vi "Do_Every_minute.vi"(1 "Ch Names":string[](array[string]), 2 "Values":dbl[](array[numeric]) format="%.2f") -> ()   [LabVIEW 2011]
uses:
  Do_Every_5mins.ctl
  Anemometry/Anemometry Sub Vis/Controls/In_Range.ctl
  ADAM Client/Sub VIs/ADAM Controls/Traverse_Level_State.ctl
  ADAM Client/Sub VIs/ADAM Controls/Valco_valve_ph.ctl
  ADAM_Global.vi
panel:
  out "Case":T1
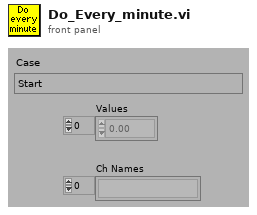
[diagram p1: front panel]
types:
  T1 = typedef "Do_Every_5mins.ctl" = enum16{"Start", "Update EnFlo Tunnel Speed Tweak", "Update Aero Tunnel Speed Tweak", "Aero Tunnel Server not live", "Are EnFlo Tun Fan Bearings too Hot?", "Check EnFlo tweak factor?", "Are Inlet Screens Blocked?", "Tweak demanded chilled water temp", "Is Dew point meter Alive?", "Condensation Occurring", "Condensation Alert", "More checks", "Set FFID Valve to Measure", "End"}
  T2 = typedef "In_Range.ctl" = enum16{"%", "±", "% & ±"}
  T3 = typedef "Traverse_Level_State.ctl" = enum16{"Running", "Complete"}
  T4 = typedef "Client_State_Cluster.ctl" = cluster{"Client Name":string, "Traverse level State":T3, "People to Email":string[], "Next Contact Time":dbl}
  T5 = typedef "Valco_valve_ph.ctl" = u16
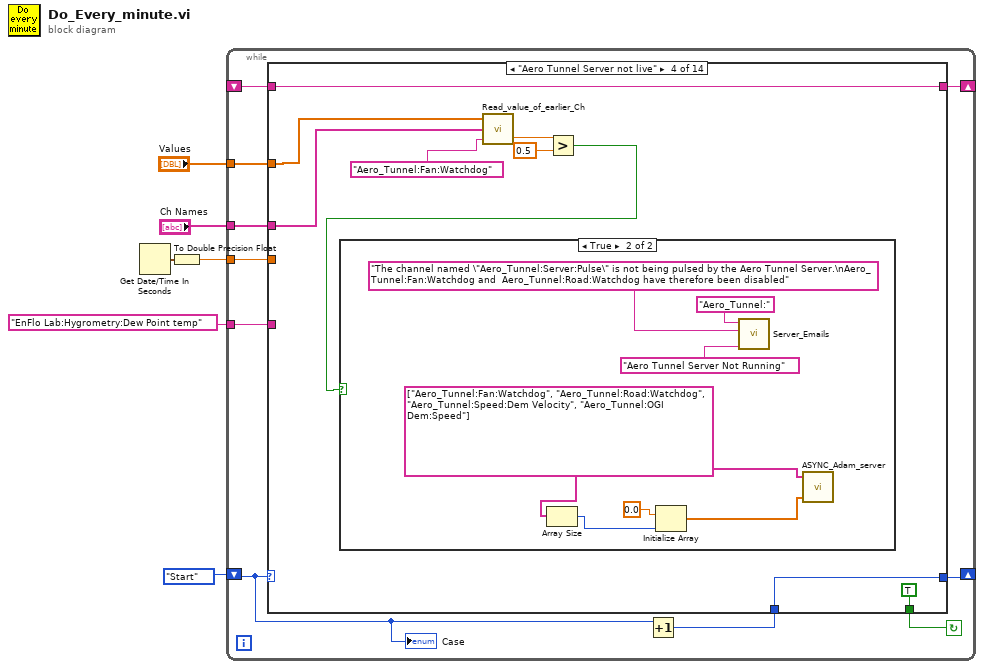
[diagram p0: block diagram]
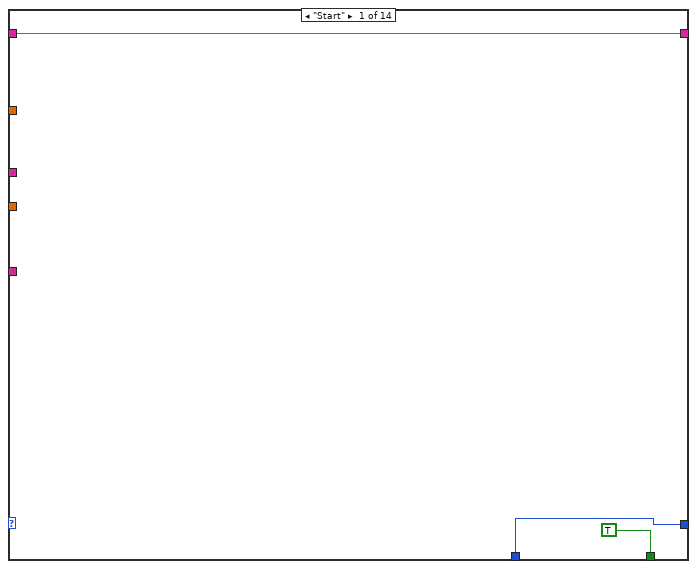
[diagram p2: hidden frame]
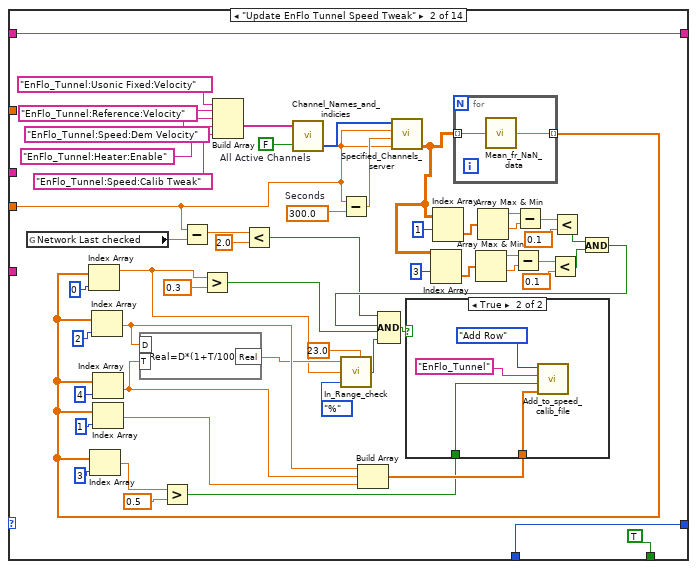
[diagram p3: hidden frame]
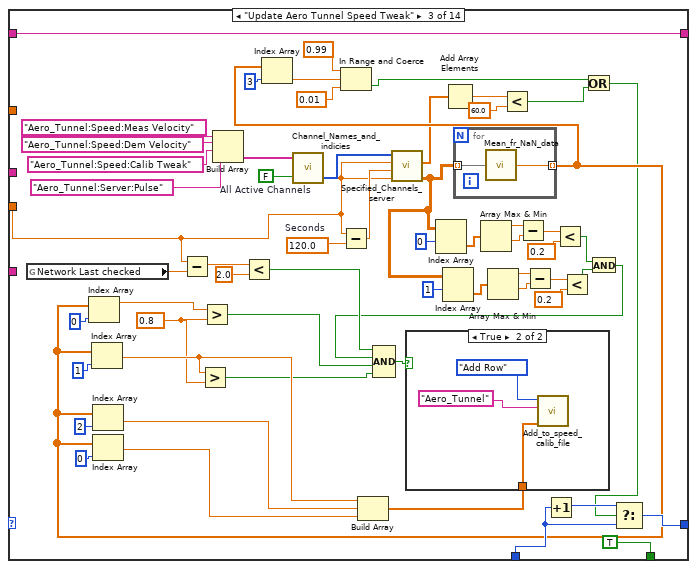
[diagram p5: hidden frame]
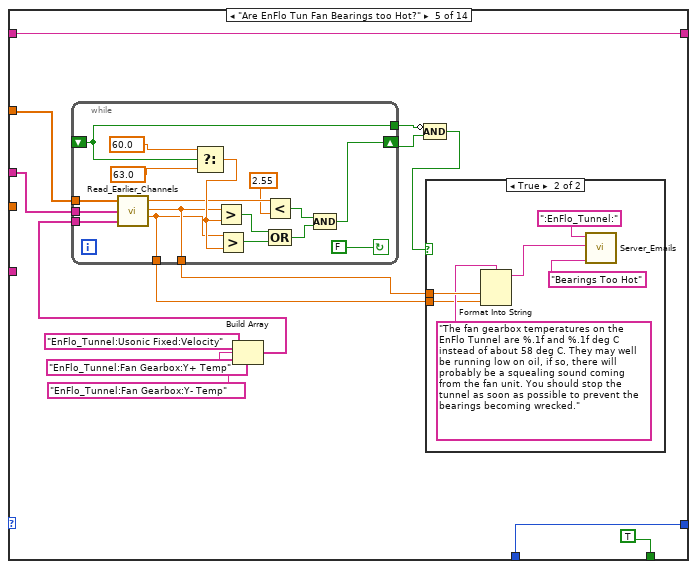
[diagram p8: hidden frame]
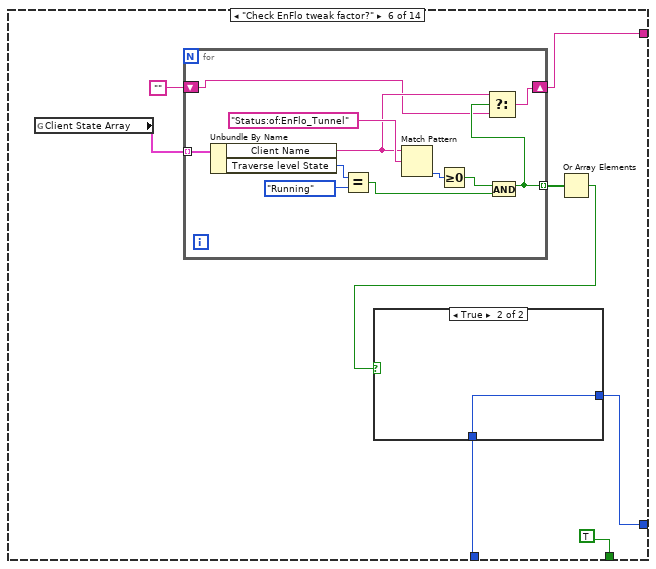
[diagram p10: hidden frame]
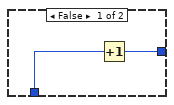
[diagram p11: hidden frame]
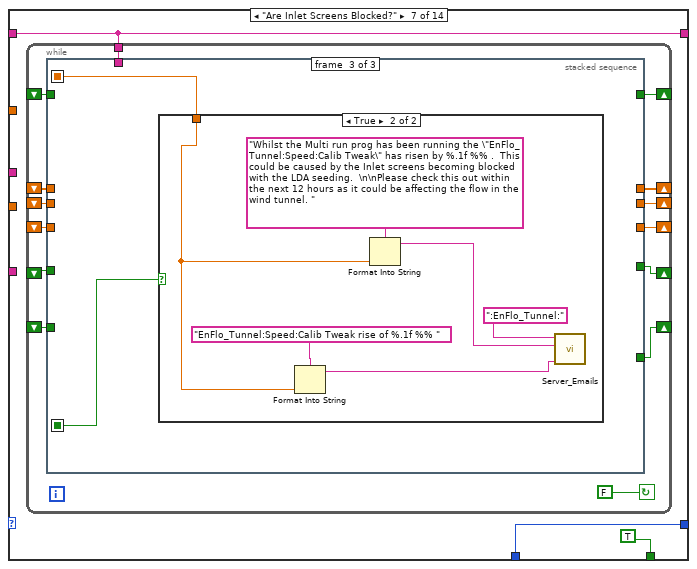
[diagram p12: hidden frame]
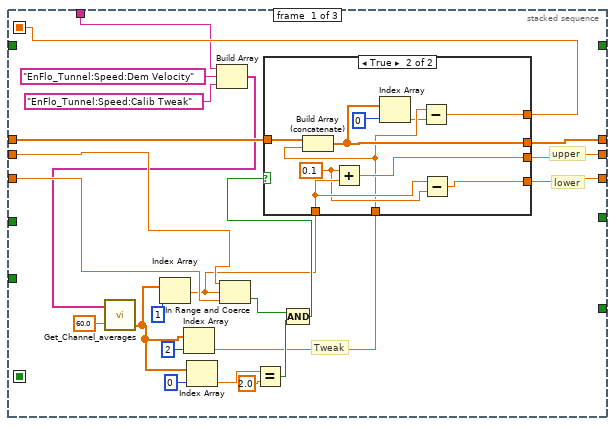
[diagram p13: hidden frame]
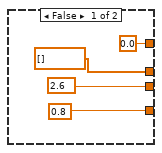
[diagram p14: hidden frame]
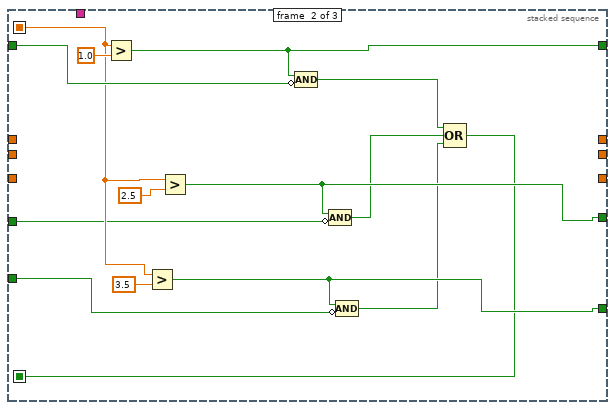
[diagram p15: hidden frame]
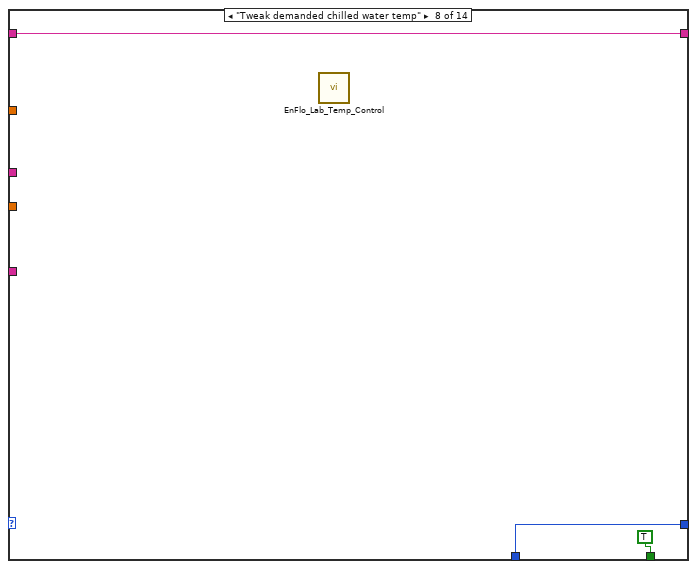
[diagram p17: hidden frame]
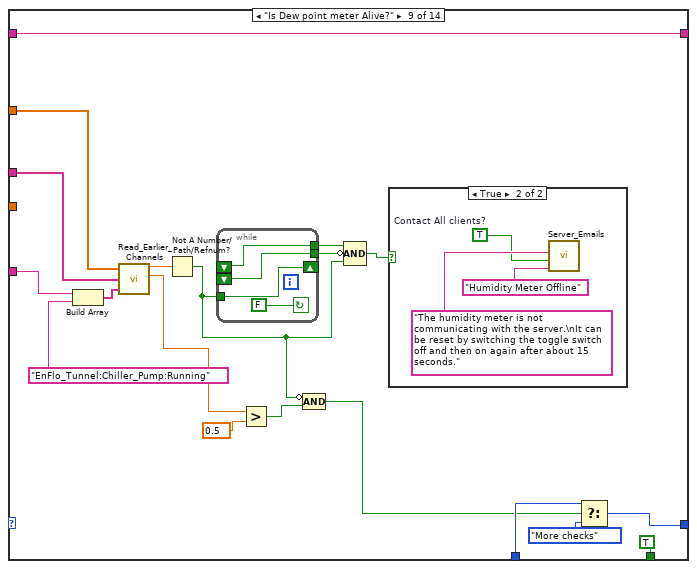
[diagram p18: hidden frame]
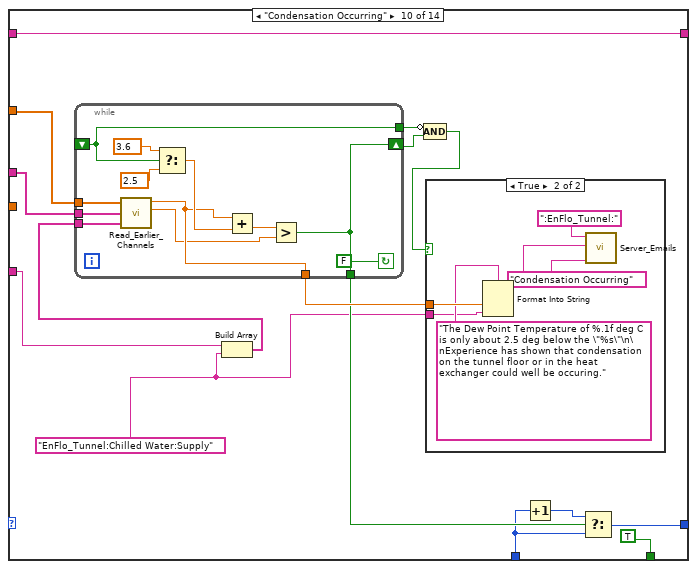
[diagram p20: hidden frame]
diagram:
  n1 = Get Date/Time In Seconds() -> (seconds since 1Jan1904=w2:timestamp)
  n2 = To Double Precision Float(number=w2) -> (double precision float=w1:dbl)
  n3 = while {
    tunnel: "EnFlo Lab:Hygrometry:Dew Point temp" -> [w10]
    tunnel: "Values" -> [w14]
    tunnel: "Ch Names" -> [w15]
    shift-left: Do_Every_5mins."Start" ("Case") -> [w11]
    shift-right: [w12] -> _
    tunnel: w1 -> [w9]
    shift-right: [w8] -> _
    shift-left: _ -> [w7]
    stop <- w16 continue-if-true
    n4 = Increment(x=w11) -> (x+1=w13:T1)
    n5 = case shown="\"Aero Tunnel Server not live\"" w11 {
      tunnel: [TRUE TRUE TRUE TRUE TRUE TRUE TRUE TRUE TRUE TRUE TRUE TRUE TRUE FALSE] -> w16
      tunnel: w15 -> [_ _ _ w148 w171 _ _ _ w313 w337 w365 w400 w404 _]
      tunnel: w14 -> [_ _ _ w149 w172 _ _ _ w314 w338 w366 w401 w403 _]
      tunnel: w13 -> [w17 w62 w90 w152 w162 w202 w221 w298 w305 w328 w368 w397 w423 w438]
      tunnel: [w17 w62 w89 w152 w162 w201 w221 w298 w317 w329 w368 w396 w423 w438] -> w12
      tunnel: w10 -> [_ _ _ _ _ _ _ _ w312 w331 w359 _ _ _]
      tunnel: w9 -> [_ w21 w111 _ _ _ _ _ _ _ _ _ w421 _]
      tunnel: [w18 w25 w115 w151 w161 w198 w220 w296 w299 w326 w358 w399 w422 w439] -> w8
      tunnel: w7 -> [w18 w25 w115 w151 w161 _ w220 w296 w299 w326 w358 w399 w422 w439]
      frame "Start" {
      }
      frame "Update EnFlo Tunnel Speed Tweak" {
        w56 = 300.0  # Seconds
        w58 = FALSE  # All Active Channels
        n6 = global read "ADAM_Global.vi" "Network Last checked"() -> (w22:dbl)
        n7 = Subtract(x=w21, y=w22) -> (x-y=w23:dbl)
        n8 = Build Array("EnFlo_Tunnel:Usonic Fixed:Velocity", "EnFlo_Tunnel:Reference:Velocity", "EnFlo_Tunnel:Speed:Dem Velocity", "EnFlo_Tunnel:Heater:Enable", "EnFlo_Tunnel:Speed:Calib Tweak") -> (w55:string[])
        n9 = Less?(x=w23, y=2.0) -> (x < y?=w20:bool)
        n10 = call "Channel_Names_and_indicies.vi"("All Active Channels"=w58, "Desired Ch Names"=w55) -> ("Indicies"=w57:i32[])  [unwired: 1 out]
        n11 = Subtract(x=w21, y=w56) -> (x-y=w54:dbl)
        n12 = call "Specified_Channels_server.vi"("End time"=w21, "Start time"=w54, "Clients time"=w21, "Requested channels"=w57) -> ("Output array"=w36:dbl[][])  [unwired: 1 in, 4 out]
        n13 = Index Array(array=w36, index (row)=3 ("Index")) -> (element=w38:dbl[])  [unwired: 1 in]
        n14 = Index Array(array=w36, index (row)=1 ("Index")) -> (element=w52:dbl[])  [unwired: 1 in]
        n15 = for {
          tunnel: w36 -> [w76] mode=indexing
          tunnel: [w75] -> w45 mode=indexing
          n16 = call "Mean_fr_NaN_data.vi"("Data"=w76) -> ("Mean value"=w75:dbl)
        }
        n17 = Index Array(array=w45, index=0) -> (element=w29:dbl)
        n18 = Index Array(array=w45, index=3) -> (element=w65:dbl)
        n19 = Index Array(array=w45, index=2) -> (element=w31:dbl)
        n20 = Index Array(array=w45, index=4) -> (element=w32:dbl)
        n21 = Index Array(array=w45, index=1) -> (element=w43:dbl)
        n22 = formula code="Real=D*(1+T/100);"("D"=w31, "T"=w32) -> ("Real"=w30:dbl)
        n23 = Greater?(x=w65, y=0.5) -> (0:w44:bool)
        n24 = Greater?(x=w29, y=0.3) -> (0:w63:bool)
        n25 = call "In_Range_check.vi"("%"=23.0, "Mode"=In_Range."%", "Value"=w29, "Setpoint"=w30) -> ("In Range"=w26:bool)  [unwired: 1 in, 2 out]
        n26 = Build Array(w31, w32, w43) -> (w60:dbl[])
        n27 = Array Max & Min(array=w38) -> (max value=w39:dbl, min value=w40:dbl)  [unwired: 2 out]
        n28 = Array Max & Min(array=w52) -> (max value=w51:dbl, min value=w50:dbl)  [unwired: 2 out]
        n29 = Subtract(x=w39, y=w40) -> (x-y=w41:dbl)
        n30 = Subtract(x=w51, y=w50) -> (x-y=w49:dbl)
        n31 = Less?(x=w41, y=0.1) -> (x < y?=w35:bool)
        n32 = Less?(x=w49, y=0.1) -> (x < y?=w34:bool)
        n33 = And(x=w34, y=w35) -> (x .and. y?=w33:bool)
        n34 = Compound Arithmetic op=AND(w20, w33, w63, w26) -> (w59:bool)
        n35 = case shown="True" w59 {
          tunnel: w60 -> [_ w79]
          tunnel: w44 -> [_ w78]
          frame False {
          }
          frame True {
            n36 = call "Add_to_speed_calib_file.vi"("New Row"=w79, "Tunnel Heated?"=w78, "Rig Name"="EnFlo_Tunnel" ("y"), "Mode"=enum16{"Add Row", "Get Error Value"}."Add Row") -> ()  [unwired: 2 in, 2 out]
          }
        }
      }
      frame "Update Aero Tunnel Speed Tweak" {
        w128 = 120.0  # Seconds
        w130 = FALSE  # All Active Channels
        w108 = 0.8 ("y")
        n37 = global read "ADAM_Global.vi" "Network Last checked"() -> (w112:dbl)
        n38 = Subtract(x=w111, y=w112) -> (x-y=w113:dbl)
        n39 = Build Array("Aero_Tunnel:Speed:Meas Velocity", "Aero_Tunnel:Speed:Dem Velocity", "Aero_Tunnel:Speed:Calib Tweak", "Aero_Tunnel:Server:Pulse") -> (w127:string[])
        n40 = Less?(x=w113, y=2.0) -> (x < y?=w110:bool)
        n41 = call "Channel_Names_and_indicies.vi"("All Active Channels"=w130, "Desired Ch Names"=w127) -> ("Indicies"=w129:i32[])  [unwired: 1 out]
        n42 = Subtract(x=w111, y=w128) -> (x-y=w126:dbl)
        n43 = call "Specified_Channels_server.vi"("End time"=w111, "Start time"=w126, "Clients time"=w111, "Requested channels"=w129) -> ("Output array"=w100:dbl[][], "Averaging Period"=w86:dbl[])  [unwired: 1 in, 3 out]
        n44 = Index Array(array=w100, index (row)=0 ("Index")) -> (element=w87:dbl[])  [unwired: 1 in]
        n45 = Index Array(array=w100, index (row)=1 ("Index")) -> (element=w102:dbl[])  [unwired: 1 in]
        n46 = Add Array Elements(numeric array=w86) -> (sum=w85:dbl)
        n47 = for {
          tunnel: w100 -> [w141] mode=indexing
          tunnel: [w140] -> w88 mode=indexing
          n48 = call "Mean_fr_NaN_data.vi"("Data"=w141) -> ("Mean value"=w140:dbl)
        }
        n49 = Index Array(array=w88, index=0) -> (element=w116:dbl)
        n50 = Index Array(array=w88, index=1) -> (element=w109:dbl)
        n51 = Index Array(array=w88, index=2) -> (element=w117:dbl)
        n52 = Index Array(array=w88, index=0) -> (element=w118:dbl)
        n53 = Greater?(x=w109, y=w108) -> (0:w107:bool)
        n54 = Greater?(x=w116, y=w108) -> (0:w134:bool)
        n55 = Index Array(array=w88, index=3) -> (element=w92:dbl)
        n56 = In Range and Coerce(upper limit=0.99, x=w92, lower limit=0.01) -> (In Range?=w82:bool)  [unwired: 1 out]
        n57 = Build Array(w109, w117, w118) -> (w132:dbl[])
        n58 = Array Max & Min(array=w87) -> (max value=w124:dbl, min value=w123:dbl)  [unwired: 2 out]
        n59 = Array Max & Min(array=w102) -> (max value=w103:dbl, min value=w104:dbl)  [unwired: 2 out]
        n60 = Less?(x=w85, y=60.0) -> (x < y?=w83:bool)
        n61 = Subtract(x=w124, y=w123) -> (x-y=w122:dbl)
        n62 = Subtract(x=w103, y=w104) -> (x-y=w105:dbl)
        n63 = Increment(x=w90) -> (x+1=w91:T1)
        n64 = Less?(x=w122, y=0.2) -> (x < y?=w99:bool)
        n65 = Less?(x=w105, y=0.2) -> (x < y?=w98:bool)
        n66 = Or(x=w82, y=w83) -> (x .or. y?=w81:bool)
        n67 = And(x=w99, y=w98) -> (x .and. y?=w97:bool)
        n68 = Compound Arithmetic op=AND(w110, w97, w134, w107) -> (w131:bool)
        n69 = case shown="True" w131 {
          tunnel: w132 -> [_ w143]
          frame False {
          }
          frame True {
            n70 = call "Add_to_speed_calib_file.vi"("New Row"=w143, "Rig Name"="Aero_Tunnel" ("y"), "Mode"=enum16{"Add Row", "Get Error Value"}."Add Row") -> ()  [unwired: 3 in, 2 out]
          }
        }
        n71 = Select(t=w91, s=w81, f=w90) -> (s? t:f=w89:T1)
      }
      frame "Aero Tunnel Server not live" {
        n72 = call "Read_value_of_earlier_Ch.vi"("Desired Ch to Read"="Aero_Tunnel:Fan:Watchdog", "Ch names"=w148, "Present scan array"=w149) -> ("Value"=w147:dbl)  [unwired: 1 in, 1 out]
        n73 = Greater?(x=w147, y=0.5) -> (0:w145:bool)
        n74 = case shown="True" w145 {
          frame False {
          }
          frame True {
            w155 = string[] ["Aero_Tunnel:Fan:Watchdog", "Aero_Tunnel:Road:Watchdog", "Aero_Tunnel:Speed:Dem Velocity", "Aero_Tunnel:OGI Dem:Speed"] ("Channel Names")
            n75 = Array Size(array=w155) -> (size(s)=w156:i32)
            n76 = Initialize Array(0.0, w156) -> (w154:dbl[])
            n77 = call "Server_Emails.vi"("Client Name Contains"="Aero_Tunnel:", "Message"="The channel named \"Aero_Tunnel:Server:Pulse\" is not being pulsed by the Aero Tunnel Server.\nAero_Tunnel:Fan:Watchdog and  Aero_Tunnel:Road:Watchdog have therefore been disabled", "Subject"="Aero Tunnel Server Not Running" ("Error Type")) -> ()  [unwired: 2 in, 3 out]
            n78 = call "ASYNC_Adam_server.vi"("Values"=w154, "Channel Names"=w155) -> ()  [unwired: 1 in, 3 out]
          }
        }
      }
      frame "Are EnFlo Tun Fan Bearings too Hot?" {
        n79 = Build Array("EnFlo_Tunnel:Usonic Fixed:Velocity", "EnFlo_Tunnel:Fan Gearbox:Y+ Temp", "EnFlo_Tunnel:Fan Gearbox:Y- Temp") -> (w170:string[])
        n80 = while {
          tunnel: [w176] -> w163
          tunnel: [w177] -> w164
          tunnel: [w186] -> w169
          shift-left: _ -> [w186]
          shift-right: [w178] -> w168
          tunnel: w170 -> [w189]
          tunnel: w171 -> [w190]
          tunnel: w172 -> [w191]
          stop <- FALSE continue-if-true
          n81 = call "Read_Earlier_Channels.vi"("Present scan array"=w191, "Ch names"=w190, "Desired Channels"=w189) -> ("Index 0"=w184:dbl, "Index 1"=w177:dbl, "Index 2"=w176:dbl)  [unwired: 3 out]
          n82 = Select(t=60.0, s=w186, f=63.0) -> (s? t:f=w185:dbl)
          n83 = Greater?(x=w177, y=w185) -> (0:w182:bool)
          n84 = Greater?(x=w176, y=w185) -> (0:w181:bool)
          n85 = Less?(x=w184, y=2.55) -> (x < y?=w180:bool)
          n86 = Compound Arithmetic op=OR(w182, w181) -> (w179:bool)
          n87 = Compound Arithmetic op=AND(w180, w179) -> (w178:bool)
        }
        n88 = Compound Arithmetic op=AND(invert w169, w168) -> (w167:bool)
        n89 = case shown="True" w167 {
          tunnel: w164 -> [_ w195]
          tunnel: w163 -> [_ w192]
          frame False {
          }
          frame True {
            n90 = Format Into String(format string="The fan gearbox temperatures on the EnFlo Tunnel are %.1f and %.1f deg C instead of about 58 deg C. They may well be running low on oil, if so, there will probably be a squealing sound coming from the fan unit. You should stop the tunnel as soon as possible to prevent the bearings becoming wrecked." ("Format String"), w195, w192) -> (resulting string=w194:string)  [unwired: 2 in, 1 out]
            n91 = call "Server_Emails.vi"("Client Name Contains"=":EnFlo_Tunnel:", "Message"=w194, "Subject"="Bearings Too Hot" ("Error Type")) -> ()  [unwired: 2 in, 3 out]
          }
        }
      }
      frame "Check EnFlo tweak factor?" {
        n92 = global read "ADAM_Global.vi" "Client State Array"() -> (w204:T4[])
        n93 = for {
          tunnel: w204 -> [w219] mode=indexing
          tunnel: [w212] -> w203 mode=indexing
          shift-right: [w210] -> w198
          shift-left: "" -> [w209]
          n94 = Unbundle By Name(w219) -> ("Client Name"=w211:string, "Traverse level State"=w218:T3)
          n95 = Equal?(x=w218, y=Traverse_Level_State."Running" ("Traverse level State")) -> (x = y?=w216:bool)
          n96 = Match Pattern(string=w211, regular expression="Status:of:EnFlo_Tunnel" ("y")) -> (offset past match=w214:i32)  [unwired: 4 out]
          n97 = Greater Or Equal To 0?(x=w214) -> (x >= 0?=w213:bool)
          n98 = And(x=w213, y=w216) -> (x .and. y?=w212:bool)
          n99 = Select(t=w211, s=w212, f=w209) -> (s? t:f=w210:string)
        }
        n100 = Or Array Elements(Boolean array=w203) -> (logical OR=w200:bool)
        n101 = case shown="True" w200 {
          tunnel: w202 -> [w207 w208]
          tunnel: [w206 w208] -> w201
          frame False {
            n102 = Increment(x=w207) -> (x+1=w206:T1)
          }
          frame True {
          }
        }
      }
      frame "Are Inlet Screens Blocked?" {
        n103 = while {
          shift-right: [w234] -> _
          shift-left: _ -> [w235]
          shift-right: [w232] -> _
          shift-left: _ -> [w230]
          shift-right: [w233] -> _
          shift-left: _ -> [w231]
          tunnel: w220 -> [w229]
          shift-right: [w228] -> _
          shift-left: _ -> [w227]
          shift-right: [w226] -> _
          shift-left: _ -> [w223]
          shift-right: [w225] -> _
          shift-left: _ -> [w224]
          stop <- FALSE continue-if-true
          n104 = stacked-sequence {
            seq-local: [w241 _ _] -> [_ w282 w289]
            seq-local: [_ w274 _] -> [_ _ w288]
            tunnel: w235 -> [w251 _ _]
            tunnel: [w250 _ _] -> w234
            tunnel: [w248 _ _] -> w233
            tunnel: [w247 _ _] -> w232
            tunnel: w231 -> [w246 _ _]
            tunnel: w230 -> [w245 _ _]
            tunnel: w229 -> [w240 _ _]
            tunnel: [_ w286 _] -> w228
            tunnel: w227 -> [_ w285 _]
            tunnel: [_ w278 _] -> w226
            tunnel: [_ w277 _] -> w225
            tunnel: w224 -> [_ w281 _]
            tunnel: w223 -> [_ w280 _]
            frame #0 {
              # "lower"
              # "upper"
              # "Tweak"
              n105 = Build Array(w240, "EnFlo_Tunnel:Speed:Dem Velocity", "EnFlo_Tunnel:Speed:Calib Tweak") -> (w237:string[])
              n106 = call "Get_Channel_averages.vi"("Desired Ch Names"=w237, "Averaging time (mins)"=60.0) -> ("number"=w256:dbl[])  [unwired: 1 in, 2 out]
              n107 = Index Array(array=w256, index=1) -> (element=w242:dbl)
              n108 = Index Array(array=w256, index=2) -> (element=w252:dbl)
              n109 = Index Array(array=w256, index=0) -> (element=w255:dbl)
              n110 = In Range and Coerce(upper limit=w246, x=w242, lower limit=w245) -> (In Range?=w243:bool)  [unwired: 1 out]
              n111 = Equal?(x=w255, y=2.0) -> (x = y?=w253:bool)
              n112 = Compound Arithmetic op=AND(w243, w253) -> (w249:bool)
              n113 = case shown="True" w249 {
                tunnel: w252 -> [_ w266]
                tunnel: w251 -> [_ w273]
                tunnel: [dbl[] [] w268] -> w250
                tunnel: [2.6 ("y") w272] -> w248
                tunnel: [0.8 ("lower limit") w271] -> w247
                tunnel: w242 -> [_ w270]
                tunnel: [0.0 w264] -> w241
                frame False {
                }
                frame True {
                  w269 = 0.1 ("x")
                  n114 = Build Array (concatenate)(w273, w266) -> (w268:dbl[])
                  n115 = Add(x=w269, y=w270) -> (x+y=w272:dbl)
                  n116 = Index Array(array=w268, index=0) -> (element=w265:dbl)
                  n117 = Subtract(x=w266, y=w265) -> (x-y=w264:dbl)
                  n118 = Subtract(x=w270, y=w269) -> (x-y=w271:dbl)
                }
              }
            }
            frame #1 {
              n119 = Greater?(x=w282, y=1.0) -> (0:w286:bool)
              n120 = Greater?(x=w282, y=3.5) -> (0:w277:bool)
              n121 = Greater?(x=w282, y=2.5) -> (0:w278:bool)
              n122 = Compound Arithmetic op=AND(w286, invert w285) -> (w279:bool)
              n123 = Compound Arithmetic op=AND(w278, invert w280) -> (w276:bool)
              n124 = Compound Arithmetic op=AND(w277, invert w281) -> (w275:bool)
              n125 = Compound Arithmetic op=OR(w279, w276, w275) -> (w274:bool)
            }
            frame #2 {
              n126 = case shown="True" w288 {
                tunnel: w289 -> [_ w291]
                frame False {
                }
                frame True {
                  n127 = Format Into String(format string="EnFlo_Tunnel:Speed:Calib Tweak rise of %.1f %% " ("Error Type"), w291) -> (resulting string=w293:string)  [unwired: 2 in, 1 out]
                  n128 = Format Into String(format string="Whilst the Multi run prog has been running the \"EnFlo_Tunnel:Speed:Calib Tweak\" has risen by %.1f %% .  This could be caused by the Inlet screens becoming blocked with the LDA seeding.  \n\nPlease check this out within the next 12 hours as it could be affecting the flow in the wind tunnel. " ("Format String"), w291) -> (resulting string=w290:string)  [unwired: 2 in, 1 out]
                  n129 = call "Server_Emails.vi"("Client Name Contains"=":EnFlo_Tunnel:", "Message"=w290, "Subject"=w293) -> ()  [unwired: 2 in, 3 out]
                }
              }
            }
          }
        }
      }
      frame "Tweak demanded chilled water temp" {
        n130 = call "EnFlo_Lab_Temp_Control.vi"() -> ()  [unwired: 1 out]
      }
      frame "Is Dew point meter Alive?" {
        n131 = Build Array(w312, "EnFlo_Tunnel:Chiller_Pump:Running") -> (w310:string[])
        n132 = call "Read_Earlier_Channels.vi"("Present scan array"=w314, "Ch names"=w313, "Desired Channels"=w310) -> ("Index 0"=w309:dbl, "Index 1"=w307:dbl)  [unwired: 4 out]
        n133 = Not A Number/Path/Refnum?(number/path/refnum=w309) -> (NaN/Path/Refnum?=w302:bool)
        n134 = while {
          tunnel: [w319] -> w300
          tunnel: [w320] -> w301
          shift-left: _ -> [w320]
          tunnel: w302 -> [w321]
          shift-left: _ -> [w319]
          shift-right: [w321] -> _
          stop <- FALSE continue-if-true
        }
        n135 = Greater?(x=w307, y=0.5) -> (0:w306:bool)
        n136 = Compound Arithmetic op=AND(invert w302, w306) -> (w303:bool)
        n137 = Compound Arithmetic op=AND(w300, invert w301, w302) -> (w315:bool)
        n138 = case shown="True" w315 {
          frame False {
          }
          frame True {
            w322 = TRUE  # Contact All clients?
            n139 = call "Server_Emails.vi"("Message"="The humidity meter is not communicating with the server.\nIt can be reset by switching the toggle switch off and then on again after about 15 seconds." ("Bundle Element"), "Contact All clients?"=w322, "Subject"="Humidity Meter Offline" ("Error Type")) -> ()  [unwired: 2 in, 3 out]
          }
        }
        n140 = Select(t=w305, s=w303, f=Do_Every_5mins."More checks" ("Case")) -> (s? t:f=w317:T1)
      }
      frame "Condensation Occurring" {
        w325 = "EnFlo_Tunnel:Chilled Water:Supply"
        n141 = Build Array(w331, w325) -> (w336:string[])
        n142 = while {
          tunnel: [w341] -> w330
          tunnel: [w343] -> w332
          tunnel: [w344] -> w335
          shift-left: _ -> [w344]
          shift-right: [w341] -> w334
          tunnel: w336 -> [w349]
          tunnel: w337 -> [w350]
          tunnel: w338 -> [w351]
          stop <- FALSE continue-if-true
          n143 = call "Read_Earlier_Channels.vi"("Present scan array"=w351, "Ch names"=w350, "Desired Channels"=w349) -> ("Index 0"=w343:dbl, "Index 1"=w342:dbl)  [unwired: 4 out]
          n144 = Select(t=3.6, s=w344, f=2.5) -> (s? t:f=w345:dbl)
          n145 = Add(x=w343, y=w345) -> (x+y=w348:dbl)
          n146 = Greater?(x=w348, y=w342) -> (0:w341:bool)
        }
        n147 = Compound Arithmetic op=AND(invert w335, w334) -> (w333:bool)
        n148 = case shown="True" w333 {
          tunnel: w332 -> [_ w355]
          tunnel: w325 -> [_ w352]
          frame False {
          }
          frame True {
            n149 = Format Into String(format string="The Dew Point Temperature of %.1f deg C is only about 2.5 deg below the \"%s\"\n\nExperience has shown that condensation on the tunnel floor or in the heat exchanger could well be occuring." ("Format String"), w355, w352) -> (resulting string=w354:string)  [unwired: 2 in, 1 out]
            n150 = call "Server_Emails.vi"("Client Name Contains"=":EnFlo_Tunnel:", "Message"=w354, "Subject"="Condensation Occurring" ("Error Type")) -> ()  [unwired: 2 in, 3 out]
          }
        }
        n151 = Increment(x=w328) -> (x+1=w327:T1)
        n152 = Select(t=w327, s=w330, f=w328) -> (s? t:f=w329:T1)
      }
      frame "Condensation Alert" {
        n153 = Build Array(w359, "EnFlo_Tunnel:Chilled Water:Dem Temp") -> (w364:string[])
        n154 = while {
          tunnel: [w372] -> w360
          tunnel: [w374] -> w363
          shift-left: _ -> [w374]
          shift-right: [w373] -> w362
          tunnel: w364 -> [w379]
          tunnel: w365 -> [w380]
          tunnel: w366 -> [w381]
          stop <- FALSE continue-if-true
          n155 = call "Read_Earlier_Channels.vi"("Present scan array"=w381, "Ch names"=w380, "Desired Channels"=w379) -> ("Index 0"=w372:dbl, "Index 1"=w371:dbl)  [unwired: 4 out]
          n156 = Select(t=4.0, s=w374, f=3.5) -> (s? t:f=w375:dbl)
          n157 = Add(x=w372, y=w375) -> (x+y=w378:dbl)
          n158 = Greater?(x=w378, y=w371) -> (0:w373:bool)
        }
        n159 = Compound Arithmetic op=AND(invert w363, w362) -> (w361:bool)
        n160 = case shown="True" w361 {
          tunnel: w360 -> [_ w384]
          frame False {
          }
          frame True {
            n161 = Format Into String(format string="The Dew Point Temperature is only about 3.5 degrees below the chilled water setpoint temperature.\n\nExperience has shown that unless the chilled water setpoint temperature is adjusted, condensation on the tunnel floor will occur if the dew point temperature (currently at %.1f degrees) rises by much more than one degree." ("Format String"), w384) -> (resulting string=w383:string)  [unwired: 2 in, 1 out]
            n162 = call "Server_Emails.vi"("Client Name Contains"=":EnFlo_Tunnel:", "Message"=w383, "Subject"="Condensation Alert" ("Error Type")) -> ()  [unwired: 2 in, 3 out]
          }
        }
      }
      frame "More checks" {
        n163 = Build Array("Fast FID:Valco Valve:Position") -> (w394:string[])
        n164 = call "Read_Earlier_Channels.vi"("Present scan array"=w401, "Ch names"=w400, "Desired Channels"=w394) -> ("Index 0"=w387:dbl)  [unwired: 5 out]
        n165 = Equal?(x=4.0, y=w387) -> (x = y?=w391:bool)
        n166 = Equal?(x=1.0, y=w387) -> (x = y?=w390:bool)
        n167 = Not A Number/Path/Refnum?(number/path/refnum=w387) -> (NaN/Path/Refnum?=w392:bool)
        n168 = Compound Arithmetic op=OR(w390, w391, w392) -> (w389:bool)
        n169 = Select(t=Do_Every_5mins."End" ("Case"), s=w389, f=w397) -> (s? t:f=w396:T1)
      }
      frame "Set FFID Valve to Measure" {
        w420 = FALSE  # All Active Channels
        n170 = Build Array("Fast FID:Valco Valve:Position") -> (w418:string[])
        n171 = call "Channel_Names_and_indicies.vi"("All Active Channels"=w420, "Desired Ch Names"=w418) -> ("Indicies"=w419:i32[])  [unwired: 1 out]
        n172 = Subtract(x=w421, y=700.0) -> (x-y=w416:dbl)
        n173 = call "Specified_Channels_server.vi"("End time"=w421, "Start time"=w416, "Clients time"=w421, "Requested channels"=w419) -> ("Output array"=w413:dbl[][])  [unwired: 1 in, 4 out]
        n174 = Index Array(array=w413, index (row)=0 ("Index")) -> (element=w409:dbl[])  [unwired: 1 in]
        n175 = Not A Number/Path/Refnum?(number/path/refnum=w409) -> (NaN/Path/Refnum?=w408:bool[])
        n176 = Or Array Elements(Boolean array=w408) -> (logical OR=w406:bool)
        n177 = Array Max & Min(array=w409) -> (max value=w411:dbl, min value=w412:dbl)  [unwired: 2 out]
        n178 = Subtract(x=w411, y=w412) -> (x-y=w410:dbl)
        n179 = Equal To 0?(x=w410) -> (x = 0?=w407:bool)
        n180 = Compound Arithmetic op=AND(w407, invert w406) -> (w405:bool)
        n181 = case shown="True" w405 {
          tunnel: w404 -> [_ w431]
          tunnel: w403 -> [_ w430]
          frame False {
          }
          frame True {
            n182 = Build Array("FFID:System:Enable") -> (w428:string[])
            n183 = call "Read_Earlier_Channels.vi"("Present scan array"=w430, "Ch names"=w431, "Desired Channels"=w428) -> ("Index 0"=w427:dbl)  [unwired: 5 out]
            n184 = Greater?(x=w427, y=0.5) -> (0:w425:bool)
            n185 = case shown="True" w425 {
              frame False {
                n186 = Build Array(0.0) -> (w433:dbl[])
                n187 = Build Array("GMU:Gas:Enable") -> (w435:string[])
                n188 = call "ASYNC_Adam_client.vi"("Values"=w433, "Channel Names"=w435) -> ()  [unwired: 2 out]
              }
              frame True {
                w436 = T5 4 items=["", "Zero Air", "Calib 1", "Calib 2", "Measure"] ("Requested Position")
                n189 = call "Fast_FID_Valve_Control.vi"("Requested Position"=w436) -> ()  [unwired: 7 out]
              }
            }
          }
        }
      }
      frame "End" {
      }
    }
    "Case" <- w11
  }
